vi "CalculateAdjQuat.vi"(10 "qb (in)":T1, 11 "qa (in)":T1) -> (3 "Quat (out)":T1)   [LabVIEW 2015]
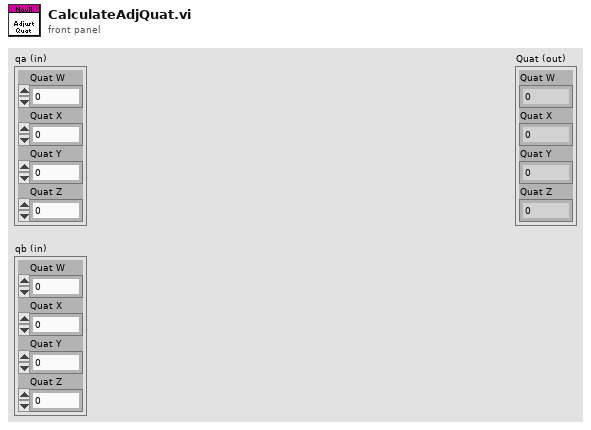
[diagram p1: front panel]
types:
  T1 = cluster{"Quat W":dbl, "Quat X":dbl, "Quat Y":dbl, "Quat Z":dbl}
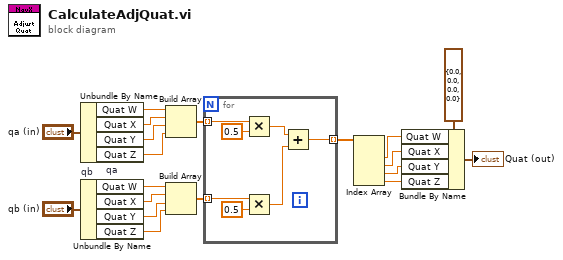
[diagram p0: block diagram]
diagram:
  n1 = Unbundle By Name "qa"("qa (in)") -> ("Quat W"=w10:dbl, "Quat X"=w11:dbl, "Quat Y"=w12:dbl, "Quat Z"=w13:dbl)
  n2 = Unbundle By Name "qb"("qb (in)") -> ("Quat W"=w14:dbl, "Quat X"=w15:dbl, "Quat Y"=w16:dbl, "Quat Z"=w17:dbl)
  n3 = Build Array(w10, w11, w12, w13) -> (w18:dbl[])
  n4 = Build Array(w14, w15, w16, w17) -> (w19:dbl[])
  n5 = for {
    tunnel: w18 -> [w26] mode=indexing
    tunnel: w19 -> [w23] mode=indexing
    tunnel: [w20] -> w6 mode=indexing
    n6 = Multiply(x=w26, y=0.5) -> (x*y=w22:dbl)
    n7 = Multiply(x=w23, y=0.5) -> (x*y=w21:dbl)
    n8 = Add(x=w22, y=w21) -> (x+y=w20:dbl)
  }
  n9 = Index Array(array=w6) -> (element #1=w5:dbl, element #2=w4:dbl, element #3=w2:dbl, element #4=w3:dbl)  [unwired: 4 in]
  n10 = Bundle By Name(cluster=T1 {"Quat W"=0.0, "Quat X"=0.0, "Quat Y"=0.0, "Quat Z"=0.0} ("Quat (out)"), "Quat W"=w5, "Quat X"=w4, "Quat Y"=w2, "Quat Z"=w3) -> (→"Quat (out)":T1)
